vi "Debug BAT_EN Startup.vi"() -> ()   [LabVIEW 2010]
uses:
  <instrlib>/Keithley 2400/Keithley 24XX.lvlib
panel:
  out "reading":dbl format="%^.2e"
  out "error out":errorcluster
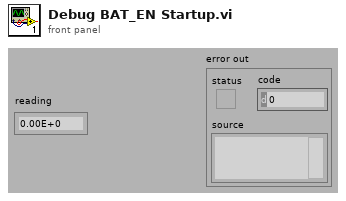
[diagram p1: front panel]
types:
  T1 = enum16{"--Disconnect All--", "Connect PulseGen to CH1", "Connect PulseGen to CH2", "Connect PulseGen to CH3", "Connect PulseGen to CH4", "Connect PulseGen to CH5", "Connect PulseGen to CH6", "Connect PulseGen to CH7", "Connect PulseGen to CH8", "Connect PulseGen to CH9", "Connect PulseGen to CH10", "Connect PulseGen to CH11", "Connect PulseGen to CH12", "Connect PulseGen to CH13", "Connect PulseGen to CH14", "Connect PulseGen to CH15", "Connect PulseGen to CH16", "Connect PulseGen to CH17", "Connect PulseGen to CH18", "Connect PulseGen to CH19", "Connect PulseGen to CH20", "Connect PulseGen to CH21", "Connect PulseGen to CH22", "Connect PulseGen to CH23", "Connect PulseGen to CH24", "Connect PulseGen to CH25", "Set MAG_SW", "Set Dynamic Load", "Set Expansion Trigger", "Trigger Positive Pulse", "Trigger Negative Pulse", "Set MSP Magic Pin", "Set BAT_EN", "Connect MSP_ACLK to CTR", "Connect MSP_MCLK to CTR", "Connect MSP_DIG_TST_OUT to CTR", "Connect STIM_SCK to CTR", "Connect STIM_CLK to CTR", "Connect SMU2 to Magnet", "Magnet Enable", "Cap Short", "Connect Positive Pulse to Pulse Bus", "Connect Negative Pulse to Pulse Bus", "Connect JTAG", "Connect JTAG DVDD Power", "RF Attach", "Connect SMU3 to VBAT", "Connect SMU3 Soft Start", "Connect ARB to Charge Coil", "Connect ARB to Matrix", "Connect CTR to Matrix", "DMM_I Short", "DMM_I 1000 Ohm", "DMM_I 100 Ohm", "DMM_I 10 Ohm", "Connect CH25 to DUT GND"}
  T2 = typedef "niSE SessionRefnum.ctl" = refnum<k1>
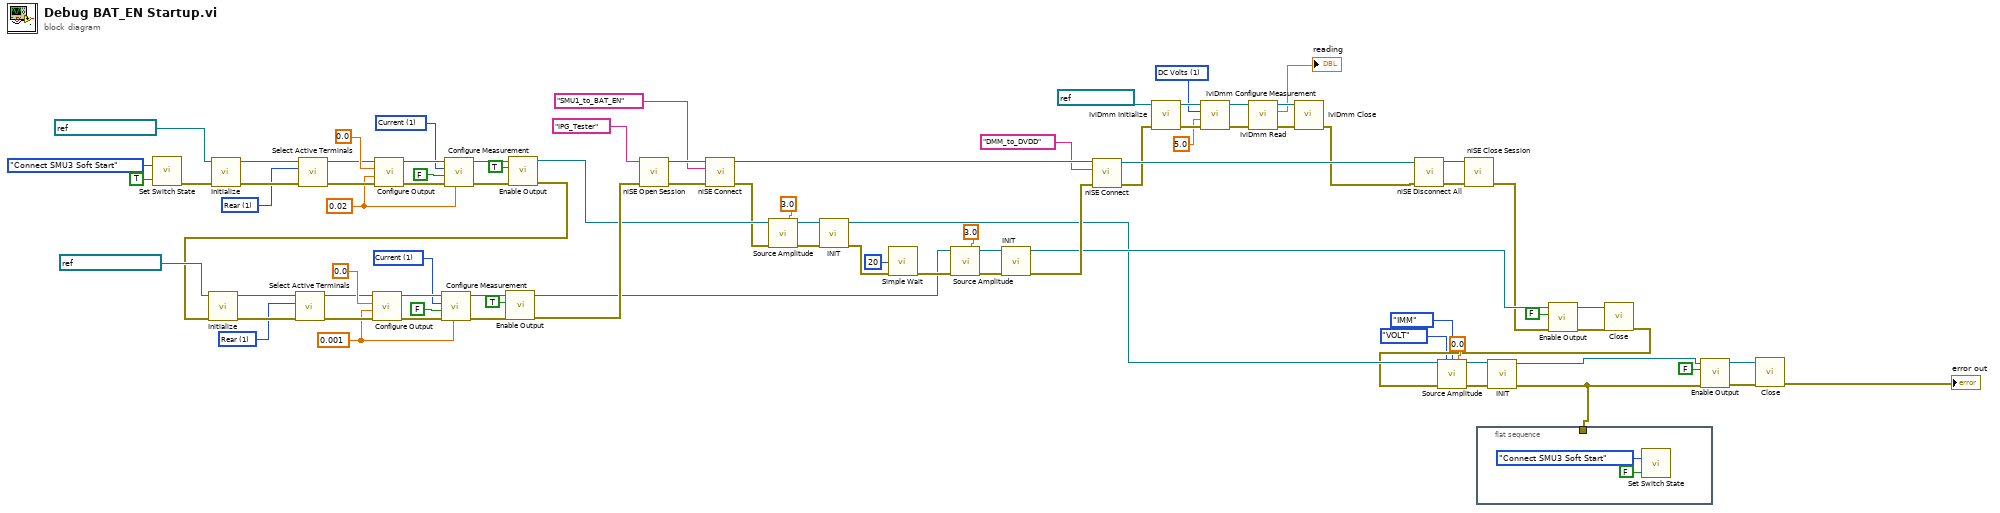
[diagram p0: block diagram]
diagram:
  w36 = u16 1 items=["Volts", "Current", "Resistance"] ("Function (0: Volts)")
  w39 = u16 1 items=["Front", "Rear"] ("Active Terminals (0: Front)")
  w15 = 0.001 ("Compliance  Level (0.1)")
  w49 = u16 1 items=["Volts", "Current", "Resistance"] ("Function (0: Volts)")
  w56 = 1 items=["DC Volts"=1, "AC Volts"=2, "DC Current"=3, "AC Current"=4, "2 Wire Resistance"=5, "4 Wire Resistance"=101, "AC + DC Volts"=106, "AC + DC Current"=107, "Frequency"=104, "Period"=105, "Temperature"=108] ("measurement function (DC Volts)")
  w64 = u16 1 items=["Front", "Rear"] ("Active Terminals (0: Front)")
  w16 = 0.02 ("Compliance  Level (0.1)")
  n1 = call "Set Switch State.vi"("Action"=T1."Connect SMU3 Soft Start", "State"=TRUE) -> ("error out"=w10:errorcluster)  [unwired: 13 in]
  n2 = call <instrlib>:"Initialize.vi"("error in (no error)"=w10, "VISA resource name"=refnum<visa-resource-name> "GPIB0::6::INSTR") -> ("error out"=w66:errorcluster, "VISA resource name out"=w68:refnum<visa-resource-name>)  [unwired: 8 in]
  n3 = call <instrlib>:"Select Active Terminals.vi"("error in (no error)"=w66, "Active Terminals (0: Front)"=w64, "VISA resource name"=w68) -> ("error out"=w65:errorcluster, "VISA resource name out"=w67:refnum<visa-resource-name>)  [unwired: 7 in]
  n4 = call <instrlib>:"Configure Output.vi"("error in (no error)"=w65, "Compliance  Level (0.1)"=w16, "Output Level (0)"=0.0, "VISA resource name"=w67) -> ("error out"=w50:errorcluster, "VISA resource name out"=w51:refnum<visa-resource-name>)  [unwired: 6 in]
  n5 = call <instrlib>:"Configure Measurement.vi"("Manual Range (1.0)"=w16, "error in (no error)"=w50, "Enable Auto Range (T:Enable)"=FALSE, "Function (0: Volts)"=w49, "VISA resource name"=w51) -> ("error out"=w46:errorcluster, "VISA resource name out"=w47:refnum<visa-resource-name>)  [unwired: 5 in]
  n6 = call <instrlib>:"Enable Output.vi"("error in (no error)"=w46, "Enable Output (T: Enable)"=TRUE, "VISA resource name"=w47) -> ("error out"=w14:errorcluster, "VISA resource name out"=w29:refnum<visa-resource-name>)  [unwired: 7 in]
  n7 = call <instrlib>:"Initialize.vi"("error in (no error)"=w14, "VISA resource name"=refnum<visa-resource-name> "GPIB0::9::INSTR") -> ("error out"=w41:errorcluster, "VISA resource name out"=w43:refnum<visa-resource-name>)  [unwired: 8 in]
  n8 = call <instrlib>:"Select Active Terminals.vi"("error in (no error)"=w41, "Active Terminals (0: Front)"=w39, "VISA resource name"=w43) -> ("error out"=w40:errorcluster, "VISA resource name out"=w42:refnum<visa-resource-name>)  [unwired: 7 in]
  n9 = call <instrlib>:"Configure Output.vi"("error in (no error)"=w40, "Compliance  Level (0.1)"=w15, "Output Level (0)"=0.0, "VISA resource name"=w42) -> ("error out"=w37:errorcluster, "VISA resource name out"=w38:refnum<visa-resource-name>)  [unwired: 6 in]
  n10 = call <instrlib>:"Configure Measurement.vi"("Manual Range (1.0)"=w15, "error in (no error)"=w37, "Enable Auto Range (T:Enable)"=FALSE, "Function (0: Volts)"=w36, "VISA resource name"=w38) -> ("error out"=w33:errorcluster, "VISA resource name out"=w34:refnum<visa-resource-name>)  [unwired: 5 in]
  n11 = call <instrlib>:"Enable Output.vi"("error in (no error)"=w33, "Enable Output (T: Enable)"=TRUE, "VISA resource name"=w34) -> ("error out"=w31:errorcluster, "VISA resource name out"=w18:refnum<visa-resource-name>)  [unwired: 7 in]
  n12 = call <vilib>:"niSE Open Session.vi"("error in (no error)"=w31, "Virtual Device Name (SwitchConfiguration1)"="IPG_Tester") -> ("error out"=w84:errorcluster, "NISE Session (out)"=w82:T2)  [unwired: 4 in]
  n13 = call <vilib>:"niSE Connect.vi"("error in (no error)"=w84, "Connection Specification (\"\")"="SMU1_to_BAT_EN" ("Connection Specification (\"\")"), "NISE Session (in)"=w82) -> ("error out"=w28:errorcluster, "NISE Session (out)"=w78:T2)  [unwired: 7 in]
  n14 = call "Source Amplitude.vi"("VISA resource name"=w29, "Source Level"=3.0, "error in (no error)"=w28) -> ("VISA resource name out"=w30:refnum<visa-resource-name>, "error out"=w27:errorcluster)  [unwired: 11 in]
  n15 = call "INIT.vi"("VISA resource name"=w30, "error in (no error)"=w27) -> ("VISA resource name out"=w6:refnum<visa-resource-name>, "error out"=w25:errorcluster)  [unwired: 12 in]
  n16 = call "Simple Wait.vi"("mS"=u32 20, "error in"=w25) -> ("error out"=w20:errorcluster)  [unwired: 12 in, 1 out]
  n17 = call "Source Amplitude.vi"("VISA resource name"=w18, "Source Level"=3.0, "error in (no error)"=w20) -> ("VISA resource name out"=w23:refnum<visa-resource-name>, "error out"=w22:errorcluster)  [unwired: 11 in]
  n18 = call "INIT.vi"("VISA resource name"=w23, "error in (no error)"=w22) -> ("VISA resource name out"=w17:refnum<visa-resource-name>, "error out"=w19:errorcluster)  [unwired: 12 in]
  n19 = call <vilib>:"niSE Connect.vi"("error in (no error)"=w19, "Connection Specification (\"\")"="DMM_to_DVDD" ("Connection Specification (\"\")"), "NISE Session (in)"=w78) -> ("error out"=w53:errorcluster, "NISE Session (out)"=w77:T2)  [unwired: 7 in]
  n20 = call <vilib>:"IviDmm Initialize.vi"("error in (no error)"=w53, "logical name (\"SampleDmm\")"=refnum<k15> "IVI-KE2000" ("logical name (\"SampleDmm\")")) -> ("error out"=w61:errorcluster, "instrument handle out"=w62:refnum<k15>)  [unwired: 8 in]
  n21 = call <vilib>:"IviDmm Configure Measurement.vi"("error in (no error)"=w61, "range (-1.0: Auto)"=5.0, "measurement function (DC Volts)"=w56, "instrument handle"=w62) -> ("error out"=w59:errorcluster, "instrument handle out"=w60:refnum<k15>)  [unwired: 6 in]
  n22 = call <vilib>:"IviDmm Read.vi"("error in (no error)"=w59, "instrument handle"=w60) -> ("error out"=w57:errorcluster, "reading"=→"reading":dbl, "instrument handle out"=w58:refnum<k15>)  [unwired: 7 in]
  n23 = call <vilib>:"IviDmm Close.vi"("error in (no error)"=w57, "instrument handle"=w58) -> ("error out"=w52:errorcluster)  [unwired: 9 in]
  n24 = call <vilib>:"niSE Disconnect All.vi"("error in (no error)"=w52, "NISE Session (in)"=w77) -> ("error out"=w83:errorcluster, "NISE Session (out)"=w81:T2)  [unwired: 4 in]
  n25 = call <vilib>:"niSE Close Session.vi"("error in (no error)"=w83, "NISE Session (in)"=w81) -> ("error out"=w13:errorcluster)  [unwired: 5 in]
  n26 = flat-sequence {
    tunnel: w3 -> [_]
    frame #0 {
      n27 = call "Set Switch State.vi"("Action"=T1."Connect SMU3 Soft Start", "State"=FALSE) -> ()  [unwired: 13 in, 1 out]
    }
  }
  n28 = call <instrlib>:"Enable Output.vi"("error in (no error)"=w13, "Enable Output (T: Enable)"=FALSE, "VISA resource name"=w17) -> ("error out"=w73:errorcluster, "VISA resource name out"=w72:refnum<visa-resource-name>)  [unwired: 7 in]
  n29 = call <instrlib>:"Close.vi"("error in (no error)"=w73, "VISA resource name"=w72) -> ("error out"=w5:errorcluster)  [unwired: 9 in]
  n30 = call "Source Amplitude.vi"("VISA resource name"=w6, "Source Function"=enum16{"CURR", "VOLT"}."VOLT", "Mode"=enum16{"IMM", "TRIGGERED"}."IMM", "Source Level"=0.0, "error in (no error)"=w5) -> ("VISA resource name out"=w9:refnum<visa-resource-name>, "error out"=w8:errorcluster)  [unwired: 9 in]
  n31 = call "INIT.vi"("VISA resource name"=w9, "error in (no error)"=w8) -> ("VISA resource name out"=w4:refnum<visa-resource-name>, "error out"=w3:errorcluster)  [unwired: 12 in]
  n32 = call <instrlib>:"Enable Output.vi"("error in (no error)"=w3, "Enable Output (T: Enable)"=FALSE, "VISA resource name"=w4) -> ("error out"=w70:errorcluster, "VISA resource name out"=w71:refnum<visa-resource-name>)  [unwired: 7 in]
  n33 = call <instrlib>:"Close.vi"("error in (no error)"=w70, "VISA resource name"=w71) -> ("error out"=→"error out":errorcluster)  [unwired: 9 in]
